vi "VI Tree.vi"   [LabVIEW 2017, in "Agilent 6000 Series.lvlib"]
doc: "This is the instrument driver for the Agilent 6000A oscilloscope series . The VI Tree displays all the user-callable VIs of the instrument driver in an organized table."
uses:
  <instrlib>/Agilent 6000 Series/Agilent 6000 Series.lvlib
  <instrlib>/Agilent 6000 Series/Public/Data/Low Data VIs/Fetch Analog Waveform.vi
  <instrlib>/Agilent 6000 Series/Public/Data/Read Single Waveform.vi
  <instrlib>/Agilent 6000 Series/Public/Configure/Configure Edge Trigger Source.vi
  <instrlib>/Agilent 6000 Series/Public/Configure/Configure Measurement Delay.vi
panel:
  # "(c) 2009-2015 National Instruments.  ALL RIGHTS RESERVED."
  # "SEE DIAGRAM\nFOR VI TREE."
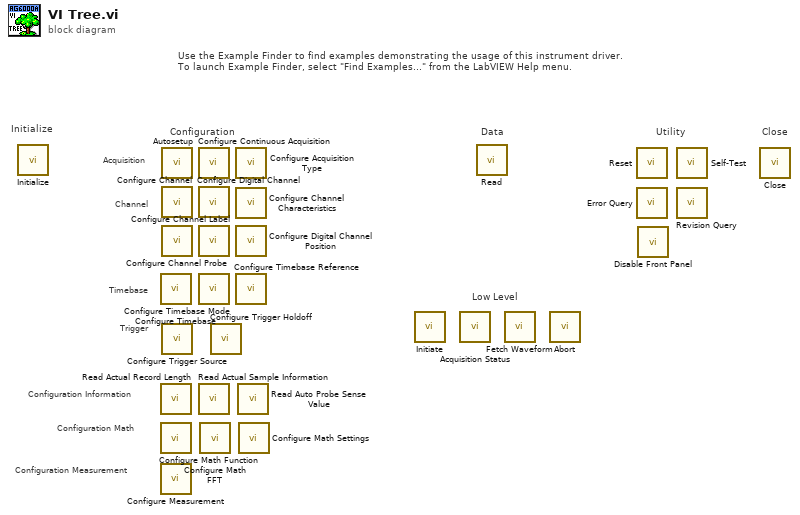
[diagram p0: block diagram]
diagram:
  # "Configuration Measurement"
  # "Configuration Math"
  # "Configuration Information"
  # "Trigger"
  # "Timebase"
  # "Acquisition"
  # "Channel"
  # "Low Level"
  # "Use the Example Finder to find examples demonstrating the usage of this instrument driver.\nTo launch Example Finder, select \"Find Examples...\" from the LabVIEW Help menu."
  # "Configuration"
  # "Utility"
  # "Data"
  # "Close"
  # "Initialize"
  n1 = call <instrlib>:"Initialize.vi"() -> ()  [unwired: 10 in, 2 out]
  n2 = call <instrlib>:"Configure Timebase.vi"() -> ()  [unwired: 10 in, 2 out]
  n3 = call <instrlib>:"Read Actual Record Length.vi"() -> ()  [unwired: 9 in, 3 out]
  n4 = call <instrlib>:"Configure Math Function.vi"() -> ()  [unwired: 10 in, 2 out]
  n5 = call-poly <instrlib>:"Configure Measurement.vi"() -> ()  [unwired: 10 in, 2 out]
  n6 = call <instrlib>:"Autosetup.vi"() -> ()  [unwired: 10 in, 2 out]
  n7 = call <instrlib>:"Configure Channel.vi"() -> ()  [unwired: 14 in, 2 out]
  n8 = call <instrlib>:"Configure Channel Probe.vi"() -> ()  [unwired: 10 in, 2 out]
  n9 = call-poly <instrlib>:"Configure Trigger Source.vi"() -> ()  [unwired: 14 in, 2 out]
  n10 = call <instrlib>:"Configure Continuous Acquisition.vi"() -> ()  [unwired: 10 in, 2 out]
  n11 = call <instrlib>:"Configure Digital Channel.vi"() -> ()  [unwired: 14 in, 2 out]
  n12 = call <instrlib>:"Configure Channel Label.vi"() -> ()  [unwired: 10 in, 2 out]
  n13 = call <instrlib>:"Configure Timebase Mode.vi"() -> ()  [unwired: 10 in, 2 out]
  n14 = call <instrlib>:"Read Actual Sample Information.vi"() -> ()  [unwired: 8 in, 4 out]
  n15 = call <instrlib>:"Configure Math FFT.vi"() -> ()  [unwired: 10 in, 2 out]
  n16 = call <instrlib>:"Configure Trigger Holdoff.vi"() -> ()  [unwired: 10 in, 2 out]
  n17 = call <instrlib>:"Configure Acquisition Type.vi"() -> ()  [unwired: 10 in, 2 out]
  n18 = call <instrlib>:"Configure Channel Characteristics.vi"() -> ()  [unwired: 10 in, 2 out]
  n19 = call <instrlib>:"Configure Digital Channel Position.vi"() -> ()  [unwired: 10 in, 2 out]
  n20 = call <instrlib>:"Configure Timebase Reference.vi"() -> ()  [unwired: 10 in, 2 out]
  n21 = call <instrlib>:"Read Auto Probe Sense Value.vi"() -> ()  [unwired: 9 in, 3 out]
  n22 = call <instrlib>:"Configure Math Settings.vi"() -> ()  [unwired: 10 in, 2 out]
  n23 = call <instrlib>:"Initiate.vi"() -> ()  [unwired: 10 in, 2 out]
  n24 = call <instrlib>:"Acquisition Status.vi"() -> ()  [unwired: 9 in, 3 out]
  n25 = call-poly <instrlib>:"Read.vi"() -> ()  [unwired: 9 in, 3 out]
  n26 = call-poly <instrlib>:"Fetch Waveform.vi"() -> ()  [unwired: 9 in, 3 out]
  n27 = call <instrlib>:"Abort.vi"() -> ()  [unwired: 10 in, 2 out]
  n28 = call <instrlib>:"Reset.vi"() -> ()  [unwired: 10 in, 2 out]
  n29 = call <instrlib>:"Error Query.vi"() -> ()  [unwired: 8 in, 4 out]
  n30 = call <instrlib>:"Disable Front Panel.vi"() -> ()  [unwired: 10 in, 2 out]
  n31 = call <instrlib>:"Self-Test.vi"() -> ()  [unwired: 8 in, 4 out]
  n32 = call <instrlib>:"Revision Query.vi"() -> ()  [unwired: 8 in, 4 out]
  n33 = call <instrlib>:"Close.vi"() -> ()  [unwired: 11 in, 1 out]
